vi "Plot Bezier Spline.vi"() -> ()   [LabVIEW 2019]
panel:
  out "bezier spline":cluster{"x":dbl, "y":dbl}[](array[cluster])
  out "Spline Graph 2":cluster{"x":dbl, "y":dbl}[](graph)
  out "Waveform Graph 3":dbl[](graph)
  out "Waveform Graph 2":dbl[](graph)
  out "Waveform Graph":dbl[](graph)
  in  "Limits":T1={"Velocity (fps)"=5.0, "Accel (fps^2)"=10.0, "Jerk (fps^3)"=100.0}
  out "l total":dbl
  out "l":dbl[](array[numeric])
  in  "ending orientation":dbl=nan
  out "curvature time":u32
  out "Spline Graph":T2(graph)
  out "Curvature":dbl[](graph)
  out "spline time":u32
  in  "percision":dbl=0.01
  in  "starting orientation":dbl
  in  "waypoints":cluster{dbl, dbl}[](array[cluster])
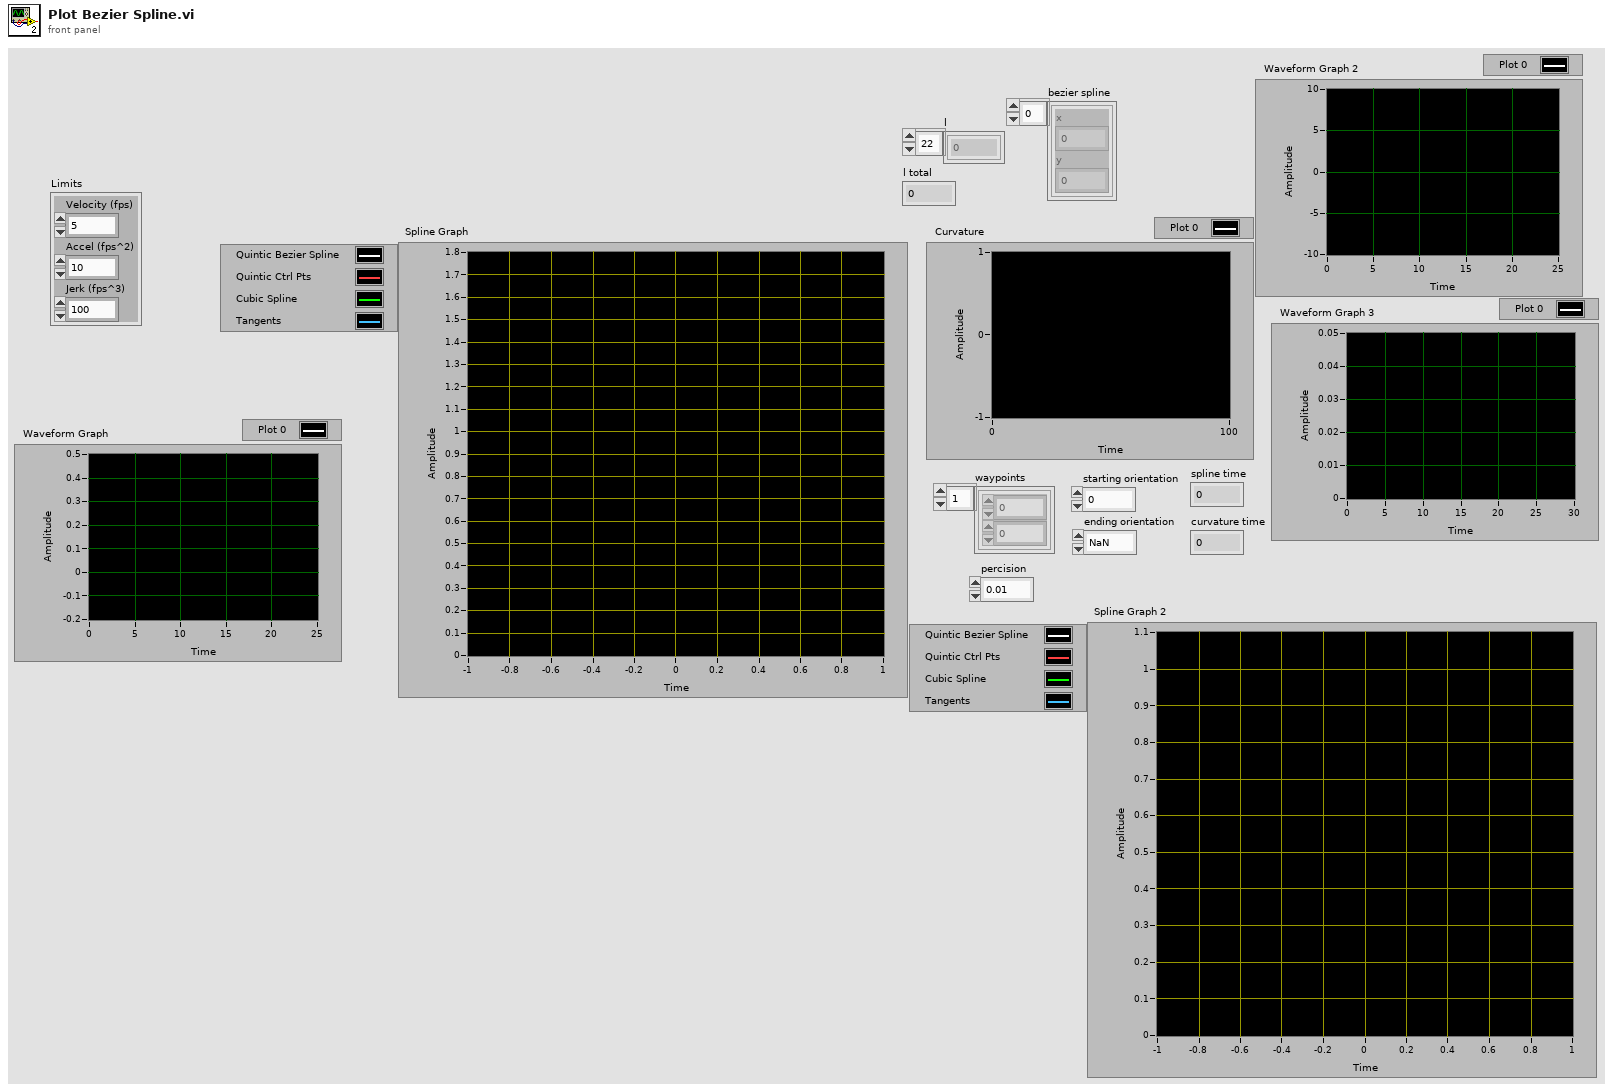
[diagram p1: front panel]
types:
  T1 = cluster{"Velocity (fps)":dbl, "Accel (fps^2)":dbl, "Jerk (fps^3)":dbl}
  T2 = cluster{"ctrl pts":cluster{"x":dbl, "y":dbl}[]}[]
  T3 = typedef "Bezier Spline.ctl" = cluster{"x":dbl, "y":dbl}[][]
  T4 = typedef "Bezier Curve.ctl" = cluster{"x":dbl, "y":dbl}[]
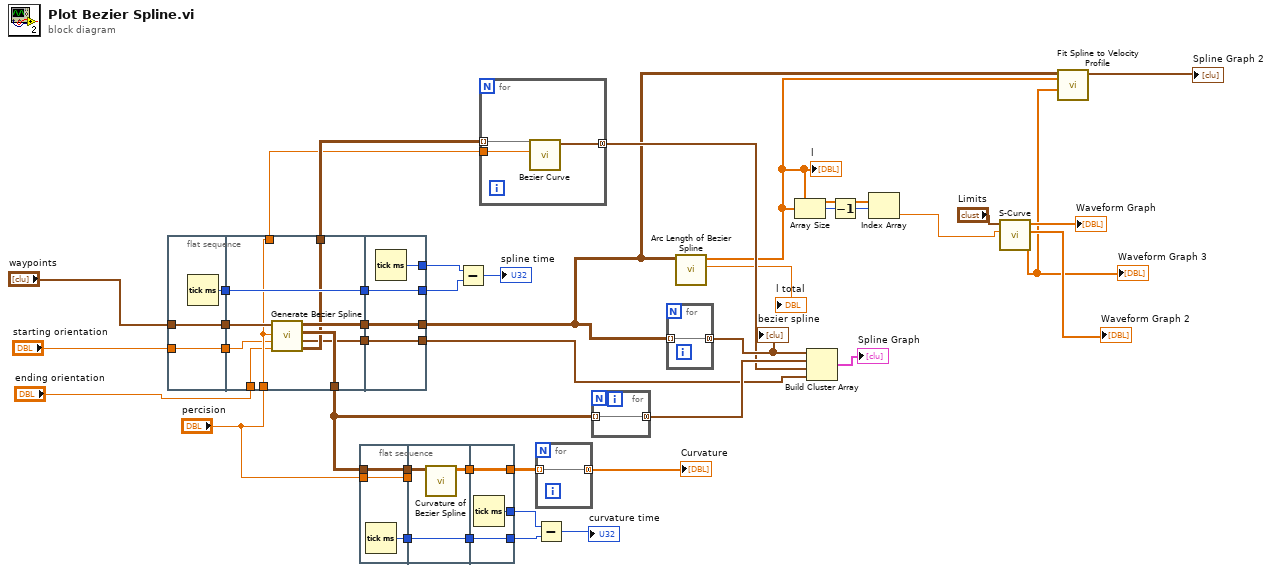
[diagram p0: block diagram]
diagram:
  n1 = flat-sequence {
    tunnel: [w45] -> w39
    tunnel: [w44] -> w37
    tunnel: "waypoints" -> [w44]
    tunnel: [w43] -> w36
    tunnel: "starting orientation" -> [w43]
    tunnel: [w54] -> w40
    tunnel: w39 -> [w54]
    tunnel: w37 -> [w53]
    tunnel: w36 -> [w47]
    tunnel: "percision" -> [w48]
    tunnel: [w52] -> w34
    tunnel: [w51] -> w30
    tunnel: [w50] -> w26
    tunnel: [w48] -> w25
    tunnel: [w49] -> w13
    tunnel: "ending orientation" -> [w46]
    tunnel: [w58] -> w42
    tunnel: [w57] -> w41
    tunnel: w40 -> [w57]
    tunnel: [w56] -> w7
    tunnel: w34 -> [w56]
    tunnel: [w55] -> w14
    tunnel: w13 -> [w55]
    frame #0 {
      n2 = Tick Count (ms)() -> (millisecond timer value=w45:u32)
    }
    frame #1 {
      n3 = call "Generate Bezier Spline.vi"("ending orientation"=w46, "starting orientation"=w47, "percision"=w48, "waypoints"=w53) -> ("cubic spline ctrl pts"=w50:cluster{dbl, dbl}[][], "Tangents"=w49:cluster{dbl, dbl}[], "ctrl pts"=w51:cluster{dbl, dbl}[][], "bezier spline"=w52:T3)  [unwired: 4 in]
    }
    frame #2 {
      n4 = Tick Count (ms)() -> (millisecond timer value=w58:u32)
    }
  }
  n5 = flat-sequence {
    tunnel: w30 -> [w60]
    tunnel: "percision" -> [w61]
    tunnel: [w61] -> w21
    tunnel: [w60] -> w20
    tunnel: [w59] -> w16
    tunnel: [w64] -> w22
    tunnel: w21 -> [_]
    tunnel: w20 -> [w63]
    tunnel: [w62] -> w17
    tunnel: w16 -> [w62]
    tunnel: [w67] -> w31
    tunnel: w22 -> [w67]
    tunnel: [w66] -> w19
    tunnel: [w65] -> w18
    tunnel: w17 -> [w65]
    frame #0 {
      n6 = Tick Count (ms)() -> (millisecond timer value=w59:u32)
    }
    frame #1 {
      n7 = call "Curvature of Bezier Spline.vi"("bezier spline waypts"=w63) -> ("curvature"=w64:dbl[][])  [unwired: 10 in]
    }
    frame #2 {
      n8 = Tick Count (ms)() -> (millisecond timer value=w66:u32)
    }
  }
  n9 = Subtract(x=w42, y=w41) -> (x-y=→"spline time":u32)
  n10 = for {
    tunnel: w26 -> [w70] mode=indexing
    tunnel: w25 -> [w69]
    tunnel: [w68] -> w24 mode=concatenating
    n11 = call "Bezier Curve.vi"("percision"=w69, "ctrl points"=w70) -> ("curve"=w68:T4)  [unwired: 9 in]
  }
  n12 = for {
    tunnel: [w71] -> w23 mode=concatenating
    tunnel: w31 -> [w71] mode=indexing
  }
  "Curvature" <- w23
  n13 = Subtract(x=w19, y=w18) -> (x-y=→"curvature time":u32)
  n14 = for {
    tunnel: [w72] -> w28 mode=concatenating
    tunnel: w30 -> [w72] mode=indexing
  }
  n15 = for {
    tunnel: w7 -> [w73] mode=indexing
    tunnel: [w73] -> w29 mode=concatenating
  }
  "bezier spline" <- w29
  n16 = call "Arc Length of Bezier Spline.vi"("bezier spline"=w7) -> ("l total"=→"l total":dbl, "l"=w2:dbl[])  [unwired: 9 in]
  "l" <- w2
  n17 = Array Size(array=w2) -> (size(s)=w4:i32)
  n18 = Build Cluster Array(w29, w28, w24, w14) -> (→"Spline Graph":cluster{"curve ":T4}[])
  n19 = Decrement(x=w4) -> (x-1=w3:i32)
  n20 = Index Array(array=w2, index=w3) -> (element=w1:dbl)
  n21 = call "S-Curve.vi"("goal"=w1, "Limits"="Limits") -> ("X"=w6:dbl[], "A"=→"Waveform Graph 2":dbl[], "V"=→"Waveform Graph":dbl[])  [unwired: 6 in, 1 out]
  "Waveform Graph 3" <- w6
  n22 = call "Fit Spline to Velocity Profile.vi"("X"=w6, "positions"=w2, "bezier spline"=w7) -> ("spline adj"=→"Spline Graph 2":cluster{"x":dbl, "y":dbl}[])  [unwired: 8 in]
